vi "lowLevelControllerRun.vi"(8 "error in (no error)":errorcluster) -> (0 "error out":errorcluster)   [LabVIEW 2017, in "lowLevelController.lvlib"]
uses:
  lowLevelController.lvlib
  UEFGV/Type Def/UEFGV_States.ctl
  TypeDefs/LoopStates.ctl
  Admittance Controller/Controls/AdmittanceGains.ctl
  <vilib>/FPGAPlugInAG/myRIO-1900/niLvFpga_Open_myRIO-1900.vi
  <vilib>/rvi/interface/common/dynamic/niFpgaDynamicAddResources.vi
  <vilib>/Utility/error.llb/Error Cluster From Error Code.vi
  <vilib>/rvi/errors/niLvFpgaAdjustHostInterfaceError.vi
  <vilib>/FPGAPlugInAG/Dynamic/niLvFpga_Close_Dynamic.vi
  <vilib>/rvi/interface/nirviOpenFPGA/nirviOpenFPGA.xnode
  FPGA Bitfiles/MyPamRefactored_FPGATarget_FPGATopLevel_TMoJaSTHfG0.lvbitx
  FPGA/FPGA Top Level.vi
  <vilib>/rvi/interface/nirviReadWriteControl/nirviReadWriteControl.xnode
  <vilib>/rvi/interface/nirviCloseFPGA/nirviCloseFPGA.xnode
  loggingModule/loggingModule.lvlib
  ErrorMonitor/ErrorMonitor.lvlib
  NiFpgaLv.dll
  <vilib>/rvi/interface/Simulation/niFpgaSimulationCallBeginRW.vi
  Admittance Controller/admittanceControllerLibrary.lvlib
panel:
  out "shutdown":bool
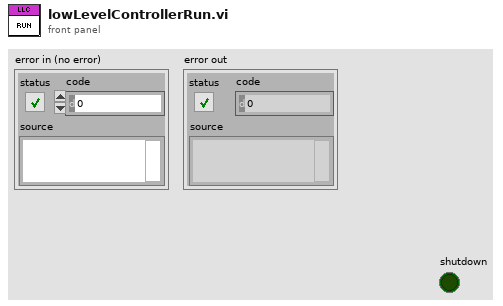
[diagram p1: front panel]
types:
  T1 = typedef "UEFGV_States.ctl" = enum16{"Create", "Get", "Destroy"}
  T2 = typedef "LoopStates.ctl" = enum16{"start", "wait", "run", "end"}
  T3 = typedef "admittanceControllerLibrary.lvlib/AdmittanceGains.ctl" = cluster{"C":dbl, "k":dbl}
  T4 = cluster{"proportional gain (Kc)":dbl, "integral time (Ti, min)":dbl, "derivative time (Td, min)":dbl}
  T5 = typedef "allData.ctl" = cluster{"DataOut":T6, "DataIn":T7}
  T6 = typedef "dataOut.ctl" = cluster{"X0pos":dbl, "Y0pos":dbl, "Z0pos":dbl, "Fx":dbl, "Fy":dbl, "Fz":dbl, "Encoder1":i32, "Encoder2":i32, "Pot1":dbl, "Pot2":dbl, "Theta0":dbl, "Theta1":dbl, "X1pos":dbl, "Y1pos":dbl, "Z1pos":dbl, "X2pos":dbl, "Y2pos":dbl, "Z2pos":dbl, "ErrorOccurred":bool}
  T7 = typedef "dataIn.ctl" = cluster{"Xtarget":dbl, "Ytarget":dbl, "Ztarget":dbl, "X_Attractor1":dbl, "Y_Attractor1":dbl, "Z_Attractor1":dbl, "X_Attractor2":dbl, "Y_Attractor2":dbl, "Z_Attractor2":dbl, "Traj_Flag":bool, "DeadZone":dbl, "Assistance":bool, "Shutdown":bool, "AssistanceLevel":dbl}
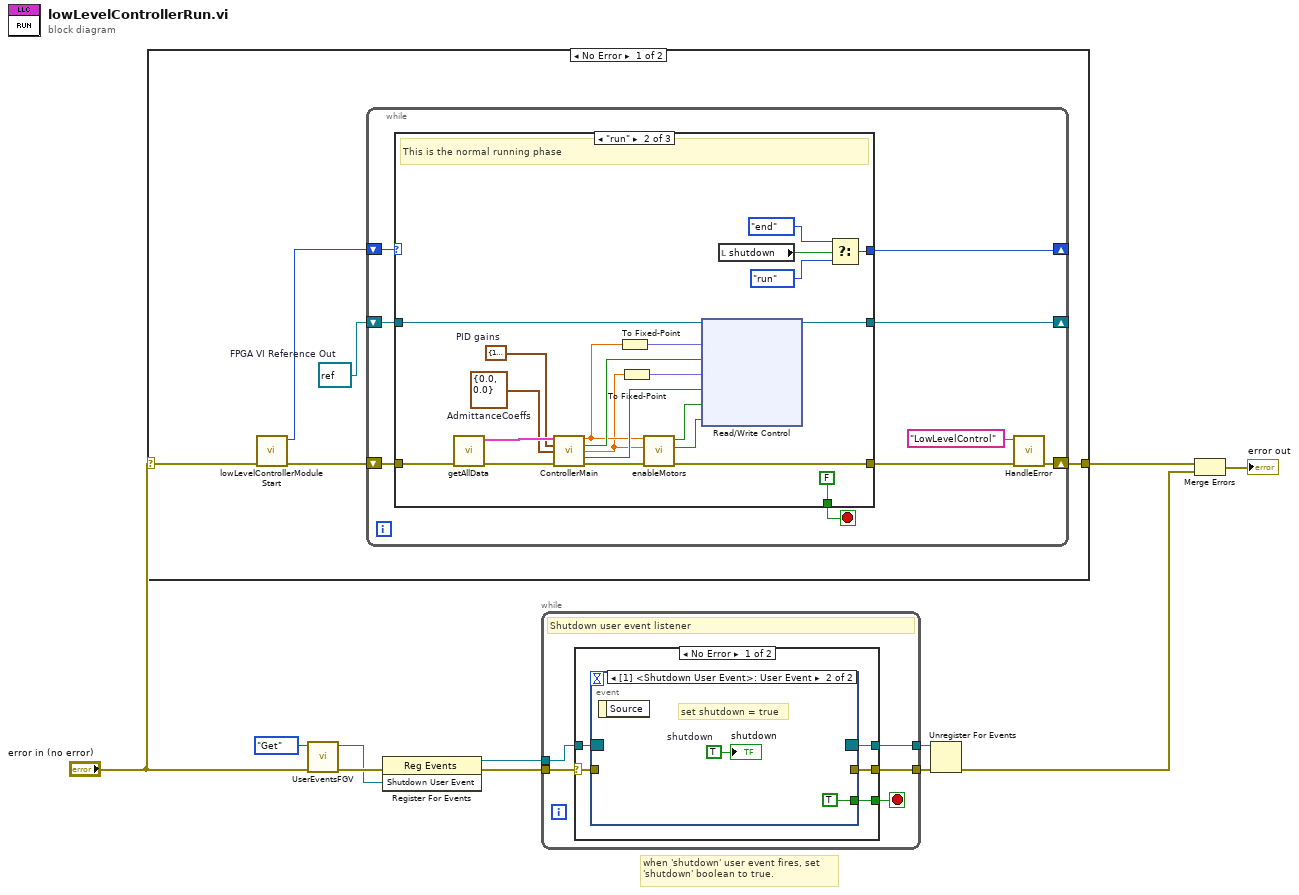
[diagram p0: block diagram]
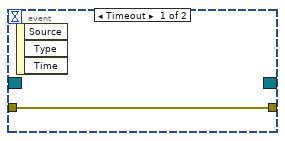
[diagram p2: hidden frame]
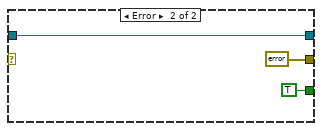
[diagram p3: hidden frame]
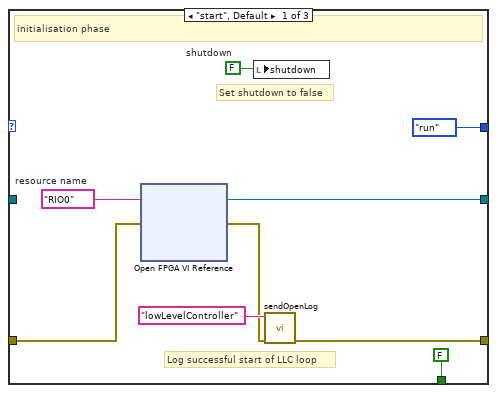
[diagram p4: hidden frame]
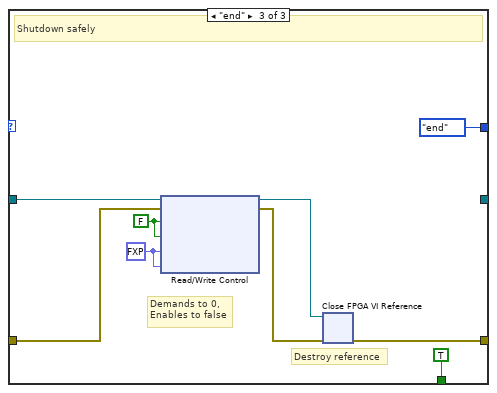
[diagram p5: hidden frame]
diagram:
  # "when 'shutdown' user event fires, set\n'shutdown' boolean to true."
  n1 = case shown="No Error" "error in (no error)" {
    selector: "error in (no error)" -> [w16 w66]
    tunnel: [w14 w66] -> w3
    frame No Error {
      w12 = refnum<k20> refnum  # FPGA VI Reference Out
      n2 = call "lowLevelControllerModuleStart.vi"("error in (no error)"=w16) -> ("error out"=w15:errorcluster, "message out"=w13:T2)  [unwired: 9 in]
      n3 = while {
        shift-right: [w23] -> _
        shift-left: w13 -> [w17]
        shift-right: [w19] -> _
        shift-left: w12 -> [w18]
        shift-right: [w21] -> w14
        shift-left: w15 -> [w25]
        stop <- w24 stop-if-true
        n4 = case shown="\"run\"" w17 {
          tunnel: w25 -> [w29 w51 w59]
          tunnel: [w32 w39 w63] -> w20
          tunnel: [FALSE FALSE TRUE] -> w24
          tunnel: [LoopStates."run" ("message out") w52 LoopStates."end" ("message out")] -> w23
          tunnel: [w27 w49 _] -> w19
          tunnel: w18 -> [_ w50 w62]
          frame "start", Default {
            w26 = tag "RIO0"  # resource name
            w34 = FALSE  # shutdown
            # "Log successful start of LLC loop"
            # "Set shutdown to false"
            # "initialisation phase"
            n5 = xnode "Open FPGA VI Reference"("error in"=w29, "resource name"=w26) -> ("FPGA VI Reference Out"=w27:refnum<k20>, "error out"=w28:errorcluster)
            n6 = local write "shutdown"(w34) -> ()
            n7 = call "sendOpenLog.vi"("error in (no error)"=w28, "source"="lowLevelController") -> ("error out"=w32:errorcluster)  [unwired: 9 in]
          }
          frame "run" {
            w41 = T3 {"C"=0.0, "k"=0.0}  # AdmittanceCoeffs
            w42 = T4 {"proportional gain (Kc)"=1.0, "integral time (Ti, min)"=0.01, "derivative time (Td, min)"=0.0}  # PID gains
            # "This is the normal running phase"
            n8 = call "getAllData.vi"("error in (no error)"=w51) -> ("error out"=w45:errorcluster, "AllData"=w46:T5)  [unwired: 9 in]
            n9 = call "ControllerMain.vi"("AllData"=w46, "PID gains"=w42, "AdmittanceCoeffs"=w41, "error in (no error)"=w45) -> ("U1"=w38:dbl, "Direction1"=w43:bool, "U2"=w37:dbl, "Direction 2"=w44:bool, "error out"=w40:errorcluster)  [unwired: 7 in]
            n10 = To Fixed-Point(number=w38) -> (fixed-point=w48:fxp<+/-,32,8>)  [unwired: 1 in]
            n11 = To Fixed-Point(number=w37) -> (fixed-point=w47:fxp<+/-,32,8>)  [unwired: 1 in]
            n12 = call "enableMotors.vi"("error in (no error)"=w40, "Link 2 Demand"=w37, "Link 1 Demand"=w38) -> ("error out"=w39:errorcluster, "Enable motor 2"=w35:bool, "Enable motor 1"=w36:bool)  [unwired: 6 in]
            n13 = xnode "Read/Write Control"("FPGA VI Reference In"=w50, "Link 1 Demand"=w48, "Link 1 Direction"=w43, "Link 2 Demand"=w47, "Link 2 Direction"=w44, "Enable motor 1"=w36, "Enable motor 2"=w35) -> ("FPGA VI Reference Out"=w49:refnum<k20>)  [unwired: 1 in, 1 out]
            n14 = local read "shutdown"() -> (w55:bool)
            n15 = Select(t=LoopStates."end" ("message out"), s=w55, f=LoopStates."run" ("message out")) -> (s? t:f=w52:T2)
          }
          frame "end" {
            w60 = fxp<+/-,32,8> 0.0 ("Link 1 Demand")
            w61 = FALSE ("Enable motor 1")
            # "Demands to 0,\nEnables to false"
            # "Destroy reference"
            # "Shutdown safely"
            n16 = xnode "Read/Write Control"("FPGA VI Reference In"=w62, "error in"=w59, "Enable motor 1"=w61, "Enable motor 2"=w61, "Link 1 Demand"=w60, "Link 2 Demand"=w60) -> ("FPGA VI Reference Out"=w58:refnum<k20>, "error out"=w57:errorcluster)
            n17 = xnode "Close FPGA VI Reference"("FPGA VI Reference In"=w58, "error in"=w57) -> ("error out"=w63:errorcluster)
          }
        }
        n18 = call "HandleError.vi"("error in (no error)"=w20, "Source"="LowLevelControl") -> ("error out"=w21:errorcluster)  [unwired: 9 in]
      }
    }
    frame Error {
    }
  }
  n19 = call "UserEventsFGV.vi"("error in (no error)"="error in (no error)", "Command"=UEFGV_States."Get") -> ("error out"=w9:errorcluster, "Shutdown User Event"=w8:refnum<user-event>)  [unwired: 8 in]
  n20 = register-events(error in=w9, w8) -> (reference out=w11:refnum<event-registration>, error out=w6:errorcluster)  [unwired: 1 in]
  n21 = while {
    tunnel: w11 -> [w71]
    tunnel: [w70] -> w10
    tunnel: w6 -> [w68]
    tunnel: [w67] -> w7
    stop <- w69 stop-if-true
    # "Shutdown user event listener"
    n22 = case shown="No Error" w68 {
      selector: w68 -> [w73 _]
      tunnel: w71 -> [w76 w81]
      tunnel: [w75 w81] -> w70
      tunnel: [w74 TRUE] -> w69
      tunnel: [w72 errorcluster {"status"=FALSE, "code"=0, "source"=""} ("error out")] -> w67
      frame No Error {
        n23 = event shown="[1] <Shutdown User Event>: User Event" {
          selector: w76 -> [_ _]
          dyn-events: [_ _] -> w75
          timeout: _ -> [_ _]
          tunnel: w73 -> [w77 _]
          tunnel: [w77 _] -> w72
          tunnel: [_ TRUE] -> w74
          event Timeout {
            n24 = event-data() -> ()  [unwired: 1 in, 3 out]
          }
          event User Event {
            w78 = TRUE  # shutdown
            # "set shutdown = true"
            n25 = event-data() -> ()  [unwired: 1 in, 1 out]
            "shutdown" <- w78
          }
        }
      }
      frame Error {
      }
    }
  }
  n26 = Unregister For Events(event registration refnum=w10, error in=w7) -> (error out=w2:errorcluster)
  n27 = Merge Errors(w3, w2) -> (→"error out":errorcluster)
